vi "Convert Enum.vi"(6 "Mouse Position":T1 caption="鼠标位置", 7 "User VI Ref":refnum<vi> caption="用户VI引用", 8 "Is Multi-select?":bool caption="为多选？", 9 "Remaining Items":refnum<vi>[](array[refnum]) caption="剩余项", 10 "Affected Items":T8 caption="受影响的项", 11 "Menu Refnum":refnum<k9> caption="菜单引用句柄") -> (3 "Menu Items To Add":T2[](array[typedef]) caption="待添加菜单项")   [LabVIEW 2020]
doc: "该VI属于修改LabVIEW快捷菜单部分。这是创建快捷菜单时调用的生成VI。该VI为LabVIEW输入添加到菜单的快捷菜单项。"
uses:
  <resource>/plugins/PopupMenus/support/Shortcut Menu Item Definition.ctl
  <resource>/plugins/PopupMenus/support/Transaction Control.ctl
  <resource>/plugins/PopupMenus/support/Position In Menu.ctl
  <resource>/plugins/PopupMenus/support/Relative Position.ctl
  <resource>/plugins/PopupMenus/support/Checkmark Status.ctl
  <resource>/plugins/PopupMenus/support/Enabled Menu Item Status.ctl
  Convert Enum.ctl
  <vilib>/Utility/miscctls.llb/LVPositionTypeDef.ctl
panel:
  # "弹出插件时必须遵循的规则：\n*该VI的文件名称必须与LLB的文件名称匹配－不同的只是文件扩展名。\n*VI必须禁用调试，否则它将作为插件被忽略。\n*所有菜单项的“标签后缀 + VI文件名”必须少于240个字符。\n*可从自定义类型断开连接“受影响的项”，从而加快插件的加载速度。存在该自定义类型的目的是使该VI和执行VI使用相同的类型。\n*除“受影响的项”之外，前面板上的其他所有控件都已锁定，以防被意外编辑。除“受影响的项”簇中的元素外，不要修改控件的类型或名称。\n*请参考即时帮助，了解每个控件的详细信息。"
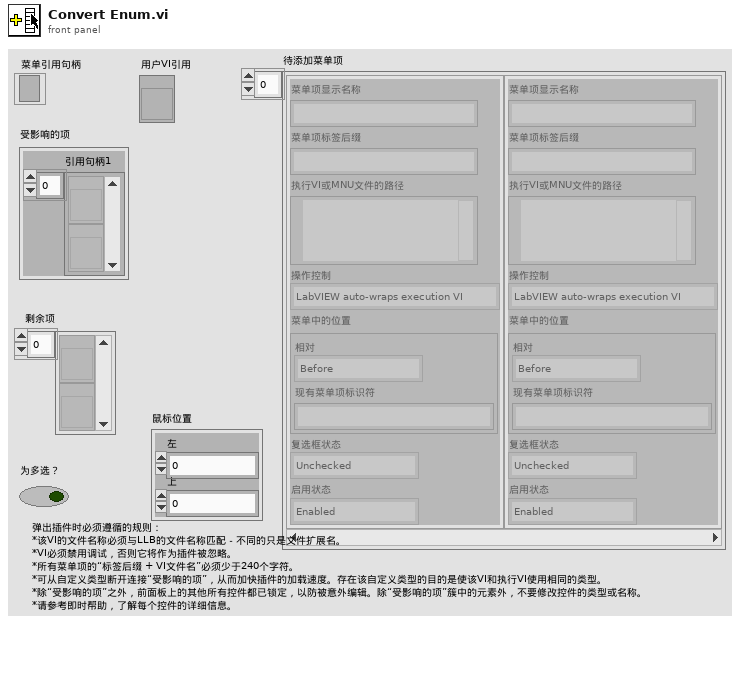
[diagram p1: front panel]
types:
  T1 = typedef "LVPositionTypeDef.ctl" = cluster{"Left":i32, "Top":i32}
  T2 = typedef "Shortcut Menu Item Definition.ctl" = cluster{"Menu Item Display Name":string, "Menu Item Tag Suffix":string, "Path To Execution VI or MNU":path, "Transaction Control":T3, "Position In Menu":T4, "Checkmark Status":T6, "Enabled Status":T7}
  T3 = typedef "Transaction Control.ctl" = enum8{"LabVIEW auto-wraps execution VI", "Execution VI will define if needed"}
  T4 = typedef "Position In Menu.ctl" = cluster{"Relative":T5, "Existing Item Tag":string}
  T5 = typedef "Relative Position.ctl" = enum8{"Before", "Instead of", "After", "Into Submenu"}
  T6 = typedef "Checkmark Status.ctl" = enum8{"Unchecked", "Checked"}
  T7 = typedef "Enabled Menu Item Status.ctl" = enum8{"Enabled", "Disabled"}
  T8 = typedef "Convert Enum.ctl" = cluster{"Refnums 1":refnum<vi>[]}
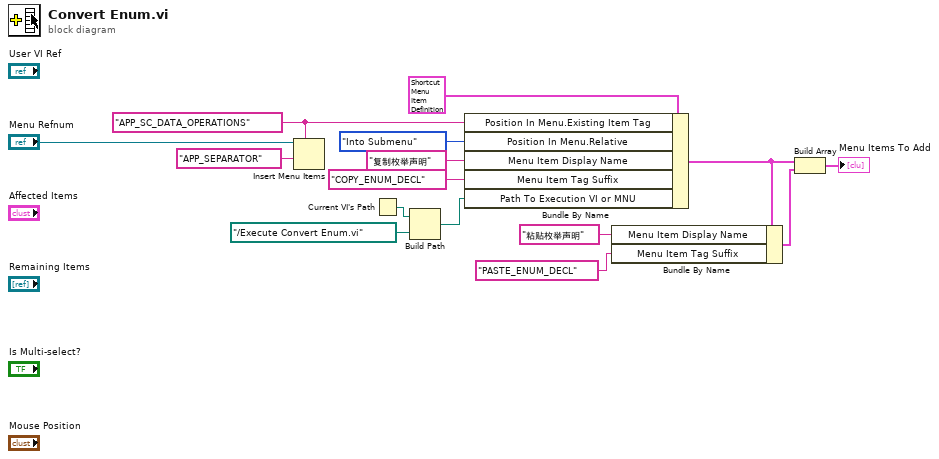
[diagram p0: block diagram]
diagram:
  w7 = "APP_SC_DATA_OPERATIONS"
  n1 = Insert Menu Items(5:w7, 7:"APP_SEPARATOR", 9:"Menu Refnum") -> ()  [unwired: 3 in, 3 out]
  n2 = Current VI's Path() -> (path=w11:path)
  n3 = Build Path(base path=w11, name or relative path=path "../Execute Convert Enum.vi" ("execute path")) -> (appended path=w14:path)
  n4 = Bundle By Name(cluster=T2 {"Menu Item Display Name"="", "Menu Item Tag Suffix"="", "Path To Execution VI or MNU"=path "", "Transaction Control"=enum."LabVIEW auto-wraps execution VI", "Position In Menu"={"Relative"=enum."Before", "Existing Item Tag"=""}, "Checkmark Status"=enum."Unchecked", "Enabled Status"=enum."Enabled"} ("Cluster"), "Position In Menu.Existing Item Tag"=w7, "Position In Menu.Relative"=Relative_Position."Into Submenu", "Menu Item Display Name"="复制枚举声明", "Menu Item Tag Suffix"="COPY_ENUM_DECL", "Path To Execution VI or MNU"=w14) -> (w5:T2)
  n5 = Bundle By Name(cluster=w5, "Menu Item Display Name"="粘贴枚举声明", "Menu Item Tag Suffix"="PASTE_ENUM_DECL") -> (w2:T2)
  n6 = Build Array(w5, w2) -> (→"Menu Items To Add":T2[])
